vi "Init Spawn.vi"(10 "Spawn":T1) -> (2 "Spawn":refnum<class "Spawn.lvclass">)   [LabVIEW 2025, in "jettl.lvlib" / "Spawn.lvlib"]
uses:
  Spawn.lvlib
  Spawn/Spawn.lvclass
  Spawn.ctl
  Attributes/Attributes/Attributes.lvclass
  Actor/Actor.lvclass
  Base Spawn/Base Spawn.lvclass
  jettl.lvlib
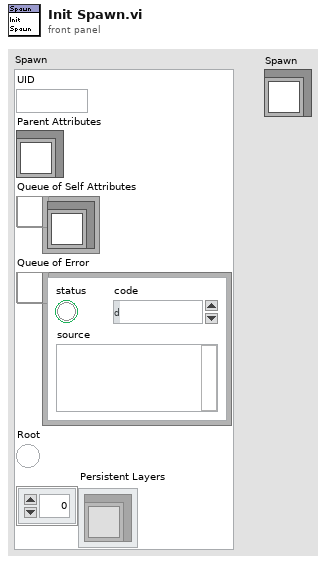
[diagram p1: front panel]
types:
  T1 = typedef "jettl.lvlib/Spawn.ctl" = cluster{"UID":string, "Parent Attributes":refnum<class "Attributes.lvclass">, "Queue of Self Attributes":refnum<queue>, "Queue of Error":refnum<queue>, "Root":bool, "Persistent Layers":refnum<class "Actor.lvclass">[]}
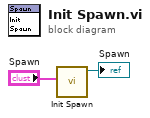
[diagram p0: block diagram]
diagram:
  n1 = call "Init Spawn.vi"("Spawn"="Spawn") -> ("Base Spawn out"=→"Spawn":refnum<class "Base Spawn.lvclass">)  [unwired: 10 in]
